vi "Get Measurement Manual Range.vi"(0 "VISA resource name":refnum<visa-resource-name>, 11 "error in (no error)":errorcluster) -> (4 "VISA resource name out":refnum<visa-resource-name>, 6 "Voltage Range out":dbl, 8 "Current Range out":dbl, 10 "Resistance Range out":dbl, 15 "error out":errorcluster)   [LabVIEW 2015, in "Keithley 2450.lvlib"]
doc: "Returns the measurement range for V, I and R on the instrument."
uses:
  <instrlib>/Keithley 2450/Keithley 2450.lvlib
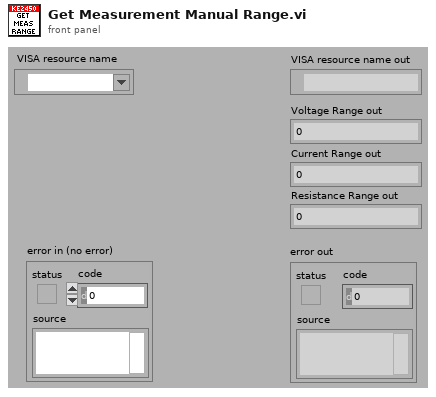
[diagram p1: front panel]
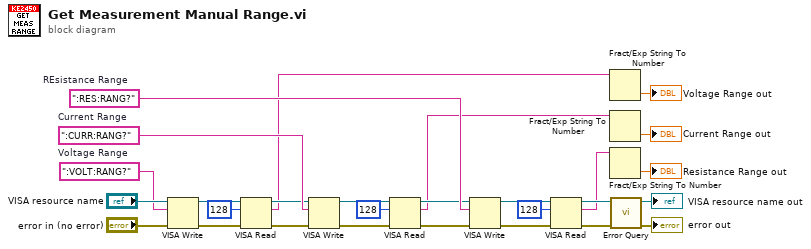
[diagram p0: block diagram]
diagram:
  w10 = ":RES:RANG?"  # REsistance Range
  w11 = ":CURR:RANG?"  # Current Range
  w12 = ":VOLT:RANG?"  # Voltage Range
  n1 = VISA Write(VISA resource name="VISA resource name", write buffer=w12, error in (no error)="error in (no error)") -> (VISA resource name out=w27:refnum<visa-resource-name>, error out=w28:errorcluster)  [unwired: 1 out]
  n2 = VISA Read(VISA resource name=w27, byte count=u32 128, error in (no error)=w28) -> (VISA resource name out=w8:refnum<visa-resource-name>, read buffer=w6:string, error out=w14:errorcluster)  [unwired: 1 out]
  n3 = VISA Write(VISA resource name=w8, write buffer=w11, error in (no error)=w14) -> (VISA resource name out=w20:refnum<visa-resource-name>, error out=w19:errorcluster)  [unwired: 1 out]
  n4 = VISA Read(VISA resource name=w20, byte count=u32 128, error in (no error)=w19) -> (VISA resource name out=w9:refnum<visa-resource-name>, read buffer=w5:string, error out=w15:errorcluster)  [unwired: 1 out]
  n5 = VISA Write(VISA resource name=w9, write buffer=w10, error in (no error)=w15) -> (VISA resource name out=w17:refnum<visa-resource-name>, error out=w18:errorcluster)  [unwired: 1 out]
  n6 = VISA Read(VISA resource name=w17, byte count=u32 128, error in (no error)=w18) -> (VISA resource name out=w7:refnum<visa-resource-name>, read buffer=w4:string, error out=w13:errorcluster)  [unwired: 1 out]
  n7 = Fract/Exp String To Number(string=w6) -> (number=→"Voltage Range out":dbl)  [unwired: 3 in, 1 out]
  n8 = Fract/Exp String To Number(string=w5) -> (number=→"Current Range out":dbl)  [unwired: 3 in, 1 out]
  n9 = Fract/Exp String To Number(string=w4) -> (number=→"Resistance Range out":dbl)  [unwired: 3 in, 1 out]
  n10 = call <instrlib>:"Error Query.vi"("error in (no error)"=w13, "VISA resource name"=w7) -> ("error out"=→"error out":errorcluster, "VISA resource name out"=→"VISA resource name out":refnum<visa-resource-name>)  [unwired: 8 out]
